vi "PutControlPlan.vi"(8 "error in (no error)":errorcluster, 10 "ControlPlan":T1, 11 "ByteGSWebAPI-V0 in":refnum<class "ByteGSWebAPI-V0.lvclass">) -> (0 "error out":errorcluster, 3 "ByteGSWebAPI-V0 out":refnum<class "ByteGSWebAPI-V0.lvclass">, 4 "body":string, 6 "headers":string)   [LabVIEW 2019, in "ByteGSWebAPI.lvlib" / "ByteGSWebAPI-V0.lvclass"]
uses:
  ByteGSWebAPI-V0.lvclass
  Cntrls/SingleControlPlan.ctl
  dbaf890d-3fd9-48d8-af77-ade9e49e7981.vi
  <vilib>/JDP Science/JSONtext/Variant to JSON Text.vi
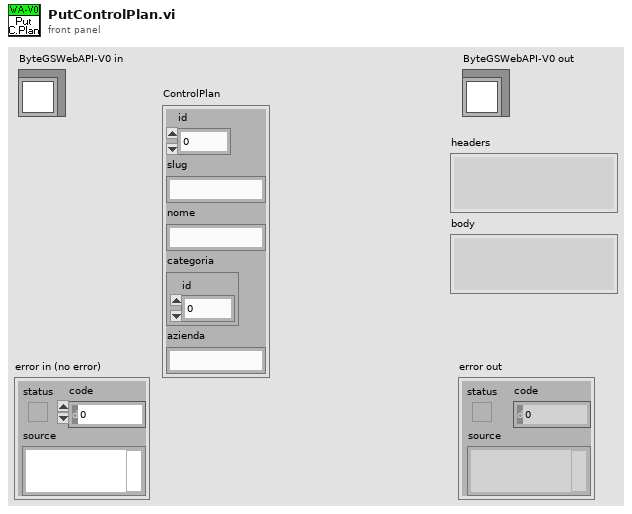
[diagram p1: front panel]
types:
  T1 = typedef "ByteGSWebAPI.lvlib/ByteGSWebAPI-V0.lvclass/SingleControlPlan.ctl" = cluster{"id":i32, "slug":string, "nome":string, "categoria":cluster{"id":i32}, "azienda":string}
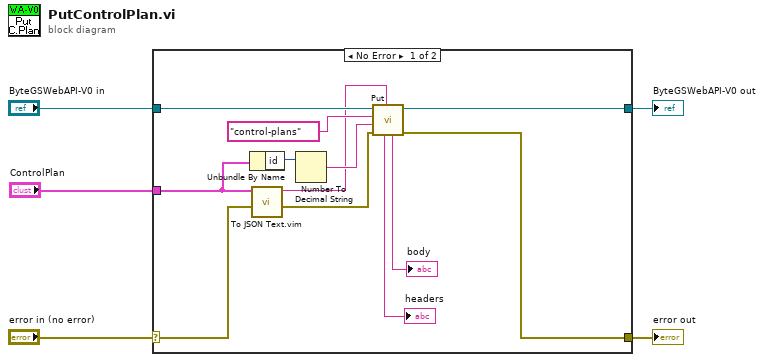
[diagram p0: block diagram]
diagram:
  n1 = case shown="No Error" "error in (no error)" {
    selector: "error in (no error)" -> [w15 w19]
    tunnel: [w8 w19] -> w4
    tunnel: [w17 w18] -> w2
    tunnel: "ByteGSWebAPI-V0 in" -> [w16 w18]
    tunnel: "ControlPlan" -> [w14 _]
    frame No Error {
      n2 = Unbundle By Name(w14) -> ("id"=w13:i32)
      n3 = call "To JSON Text.vim"("error in (no error)"=w15, "Anything"=w14) -> ("error out"=w9:errorcluster, "<JSON>"=w10:string)  [unwired: 8 in]
      n4 = Number To Decimal String(number=w13) -> (decimal integer string=w12:string)  [unwired: 1 in]
      n5 = call-dynamic "Put.vi"("PutRequest"=w10, "error in (no error)"=w9, "Parameter"=w12, "Request"="control-plans", "ByteGSWebAPI-V0 in"=w16) -> ("error out"=w8:errorcluster, "ByteGSWebAPI-V0 out"=w17:refnum<class "ByteGSWebAPI-V0.lvclass">, "body"=→"body":string, "headers"=→"headers":string)  [unwired: 3 in]
    }
    frame Error {
    }
  }
  "error out" <- w4
  "ByteGSWebAPI-V0 out" <- w2
